vi "Slider Colors Separator.vi"(8 "error in (no error)":errorcluster, 10 "Boolean":bool, 11 "NmrcWS in":refnum<class "NumericWithScale.lvclass">) -> (0 "error out":errorcluster, 3 "NmrcWS out":refnum<class "NumericWithScale.lvclass">)   [LabVIEW 2015, in "NumericWithScale.lvclass"]
uses:
  NumericWithScale.lvclass
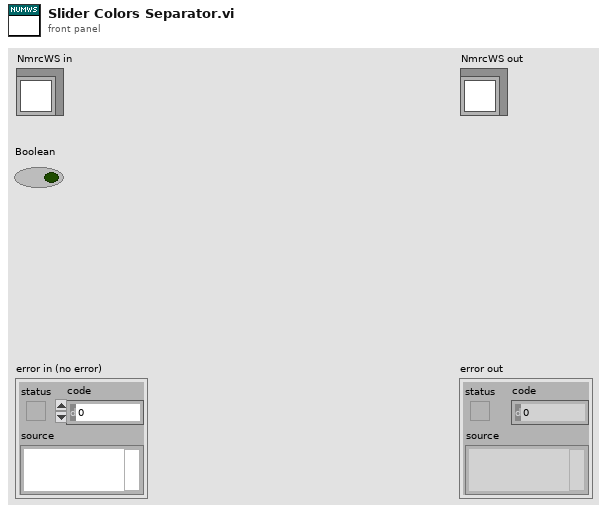
[diagram p1: front panel]
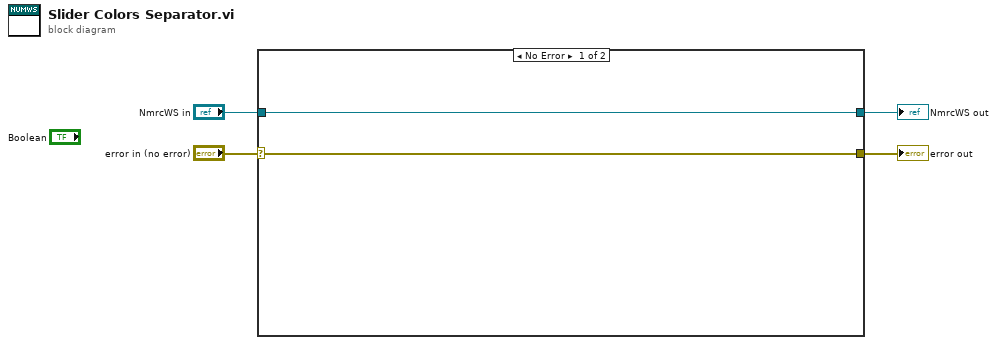
[diagram p0: block diagram]
diagram:
  n1 = case shown="No Error" "error in (no error)" {
    selector: "error in (no error)" -> [w5 w8]
    tunnel: [w5 w8] -> w3
    tunnel: [w6 w7] -> w1
    tunnel: "NmrcWS in" -> [w6 w7]
    frame No Error {
    }
    frame Error {
    }
  }
  "error out" <- w3
  "NmrcWS out" <- w1
